vi "Do.vi"(8 "error in (no error)":errorcluster, 10 "Actor in":refnum<class "Actor.lvclass">, 11 "Generate Test Event Msg":refnum<class "Generate Test Event Msg.lvclass">) -> (0 "error out":errorcluster, 2 "Actor out":refnum<class "Actor.lvclass">)   [LabVIEW 2016, in "Assert API Components.lvlib" / "Assert Display.lvlib" / "Timing Engine Tester.lvlib" / "Generate Test Event Msg.lvclass"]
doc: "This VI delivers the message to the actor by calling the appropriate method(s) on the actor."
uses:
  Generate Test Event Msg.lvclass
  <vilib>/ActorFramework/Actor/Actor.lvclass
  Timing Engine Tester/Timing Engine Tester.lvclass
  C:/Program Files (x86)/National Instruments/LabVIEW 2016/vi.lib/ActorFramework/Actor/Actor.lvclass
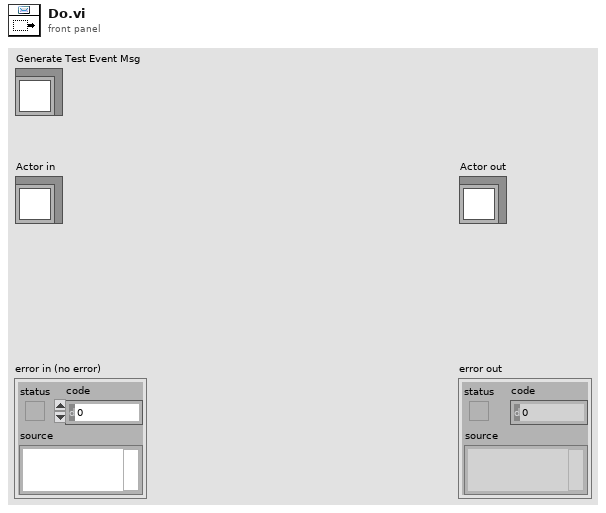
[diagram p1: front panel]
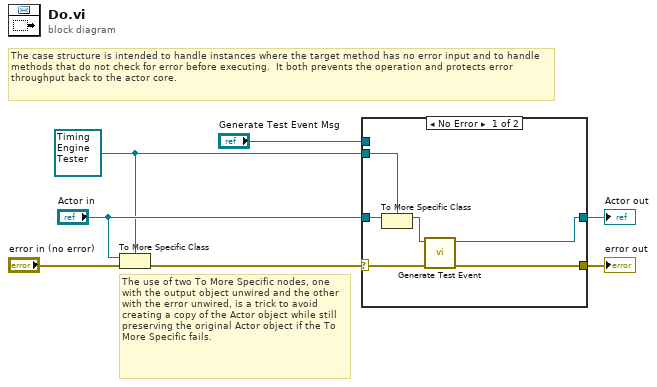
[diagram p0: block diagram]
diagram:
  w2 = refnum<class "Timing Engine Tester.lvclass"> refnum ("Actor in")
  # "The use of two To More Specific nodes, one with the output object unwired and the other with the error unwired, is a trick to avoid creating a copy of the Actor object while still preserving the original Actor object if the To More Specific fails."
  # "The case structure is intended to handle instances where the target method has no error input and to handle methods that do not check for error before executing.  It both prevents the operation and protects error throughput back to the actor core."
  n1 = To More Specific Class(target class=w2, reference="Actor in", error in="error in (no error)") -> (error out=w6:errorcluster)  [unwired: 1 out]
  n2 = case shown="No Error" w6 {
    selector: w6 -> [w11 w15]
    tunnel: [w13 w15] -> w5
    tunnel: [w12 w14] -> w4
    tunnel: "Actor in" -> [w10 w14]
    tunnel: w2 -> [w9 _]
    tunnel: "Generate Test Event Msg" -> [_ _]
    frame No Error {
      n3 = To More Specific Class(target class=w9, reference=w10) -> (specific class reference=w8:refnum<class "Timing Engine Tester.lvclass">)  [unwired: 1 in, 1 out]
      n4 = call "Generate Test Event.vi"("error in (no error)"=w11, "Timing Engine Tester in"=w8) -> ("error out"=w13:errorcluster, "Timing Engine Tester out"=w12:refnum<class "Timing Engine Tester.lvclass">)  [unwired: 8 in]
    }
    frame Error {
      # "If type check fails, pass the original object out again."
    }
  }
  "error out" <- w5
  "Actor out" <- w4
